vi "Update.vi"(8 "error in (no error)":errorcluster, 10 "Message in":refnum<class "UpdateMessage.lvclass">, 11 "ExampleClassB in":refnum<class "ExampleClassB.lvclass">) -> (0 "error out":errorcluster, 3 "ExampleClassB out":refnum<class "ExampleClassB.lvclass">)   [LabVIEW 2012, in "ExampleClassB.lvclass"]
doc: "The update method processes the command 'update'. \n\nThe command 'update' is used for receiving new values to be set to the private data of the class. This could be seen as a public set method for setting new parameters to the private class data."
uses:
  ExampleClassB.lvclass
  <vilib>/Distrio/Murmex/UpdateMessage/UpdateMessage.lvclass
  ExampleClassB.lvclass/ExampleClassB.ctl
  <vilib>/Distrio/Murmex/Murmex/status_enum.ctl
  <vilib>/Distrio/Murmex/Murmex/Murmex.lvclass
  <vilib>/Distrio/Murmex/Message/Message.lvclass
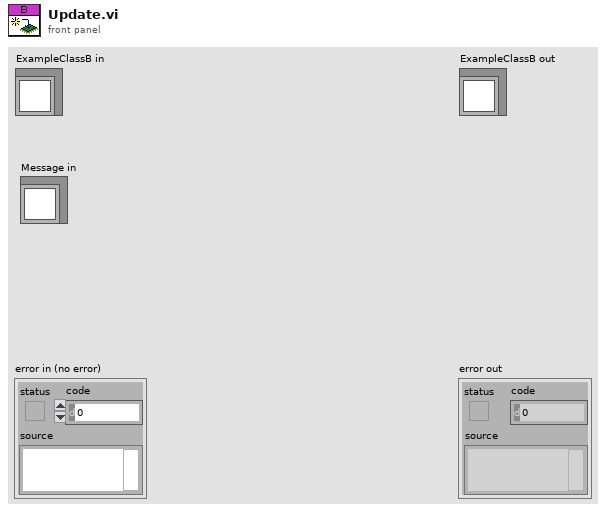
[diagram p1: front panel]
types:
  T1 = typedef "Murmex.lvlib/Murmex.lvclass/status_enum.ctl" = enum16{"ready", "warning", "error", "shutting down", "initialising"}
  T2 = typedef "ExampleClassB.lvclass/Settings cluster.ctl" = cluster{"expected samples":i32}
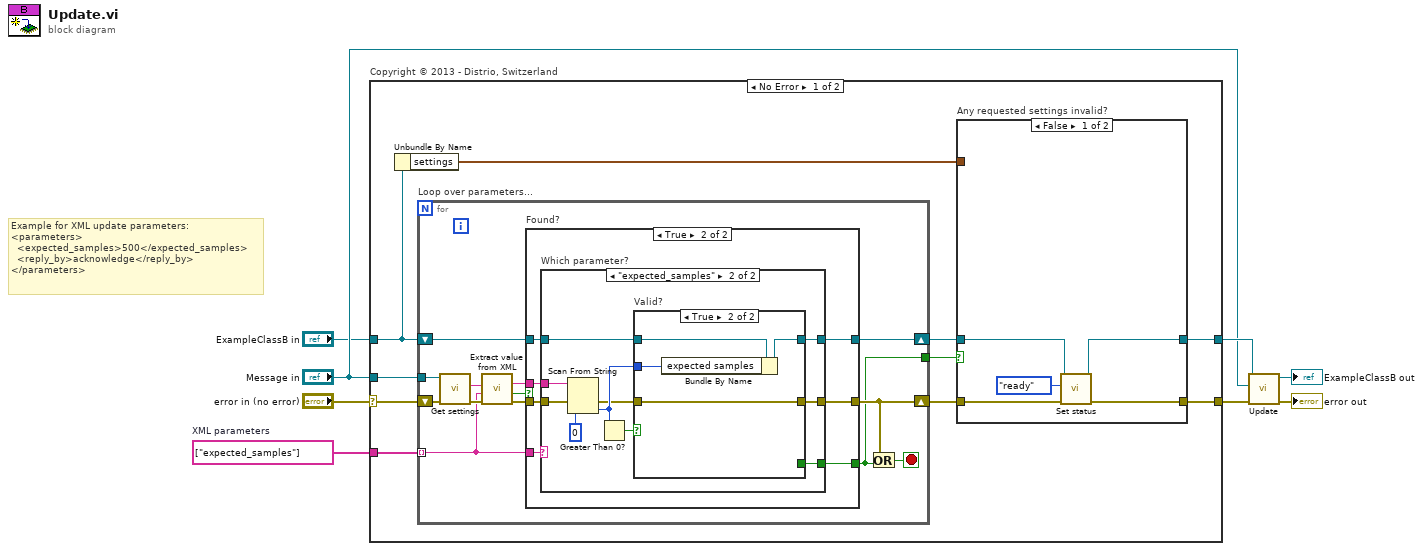
[diagram p0: block diagram]
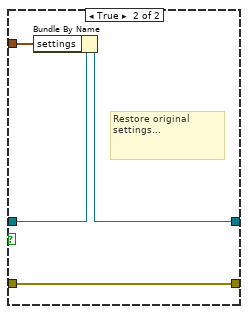
[diagram p2: hidden frame]
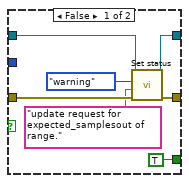
[diagram p5: hidden frame]
diagram:
  w8 = string[] ["expected_samples"]  # XML parameters
  # "Example for XML update parameters:\n<parameters>\n  <expected_samples>500</expected_samples>\n  <reply_by>acknowledge</reply_by>\n</parameters>"
  n1 = case "Copyright © 2013 - Distrio, Switzerland" shown="No Error" "error in (no error)" {
    selector: "error in (no error)" -> [w18 w73]
    tunnel: [w9 w73] -> w6
    tunnel: "ExampleClassB in" -> [w11 w74]
    tunnel: [w12 w74] -> w5
    tunnel: "Message in" -> [w17 _]
    tunnel: w8 -> [w16 _]
    frame No Error {
      n2 = Unbundle By Name(w11) -> ("settings"=w13:T2)
      n3 = for "Loop over parameters..." {
        shift-right: [w36] -> w10
        shift-left: w18 -> [w38]
        tunnel: w16 -> [w28] mode=indexing
        tunnel: w17 -> [w37]
        shift-right: [w39] -> w15
        shift-left: w11 -> [w40]
        tunnel: [w34] -> w14
        stop <- w35 stop-if-true
        n4 = call <vilib>:"Get settings.vi"("error in (no error)"=w38, "UpdateMessage in"=w37) -> ("error out"=w33:errorcluster, "settings"=w32:string)  [unwired: 7 in, 1 out]
        n5 = call <vilib>:"Extract value from XML.vi"("error in (no error)"=w33, "tag name"=w28, "parameters XML"=w32) -> ("error out"=w30:errorcluster, "found?"=w31:bool, "value"=w29:string)  [unwired: 5 in, 1 out]
        n6 = case "Found?" shown="True" w31 {
          tunnel: w30 -> [w42 w46]
          tunnel: [w42 w49] -> w36
          tunnel: w28 -> [_ w48]
          tunnel: w29 -> [_ w47]
          tunnel: w40 -> [w41 w45]
          tunnel: [w41 w44] -> w39
          tunnel: [_ w43] -> w34
          frame False {
          }
          frame True {
            n7 = case "Which parameter?" shown="\"expected_samples\"" w48 {
              tunnel: [w51 w54] -> w49
              tunnel: w47 -> [_ w57]
              tunnel: w46 -> [w51 w61]
              tunnel: w45 -> [w50 w59]
              tunnel: [w50 w58] -> w44
              tunnel: [_ w52] -> w43
              frame Default {
              }
              frame "expected_samples" {
                n8 = Scan From String(input string=w57, error in=w61, default 1=0) -> (error out=w55:errorcluster, output 1=w56:i32)  [unwired: 2 in, 2 out]
                n9 = Greater Than 0?(x=w56) -> (x > 0?=w53:bool)
                n10 = case "Valid?" shown="True" w53 {
                  tunnel: w59 -> [w68 w72]
                  tunnel: [w65 w71] -> w58
                  tunnel: w56 -> [_ w70]
                  tunnel: w55 -> [w67 w69]
                  tunnel: [w66 w69] -> w54
                  tunnel: [TRUE _] -> w52
                  frame False {
                    n11 = call <vilib>:"Set status.vi"("error in (no error)"=w67, "details"="update request for expected_samplesout of range.", "status"=status_enum."warning", "Murmex in"=w68) -> ("error out"=w66:errorcluster, "Murmex out"=w65:refnum<class "ExampleClassB.lvclass">)  [unwired: 6 in]
                  }
                  frame True {
                    n12 = Bundle By Name(cluster=w72, "expected samples"=w70) -> (w71:refnum<class "ExampleClassB.lvclass">)
                  }
                }
              }
            }
          }
        }
        n13 = Or(x=w36, y=w34) -> (x .or. y?=w35:bool)
      }
      n14 = case "Any requested settings invalid?" shown="False" w14 {
        tunnel: w15 -> [w21 w27]
        tunnel: w13 -> [_ w26]
        tunnel: [w20 w25] -> w12
        tunnel: w10 -> [w23 w24]
        tunnel: [w22 w24] -> w9
        frame False {
          n15 = call <vilib>:"Set status.vi"("error in (no error)"=w23, "status"=status_enum."ready", "Murmex in"=w21) -> ("error out"=w22:errorcluster, "Murmex out"=w20:refnum<class "ExampleClassB.lvclass">)  [unwired: 7 in]
        }
        frame True {
          # "Restore original settings..."
          n16 = Bundle By Name(cluster=w27, "settings"=w26) -> (w25:refnum<class "ExampleClassB.lvclass">)
        }
      }
    }
    frame Error {
    }
  }
  n17 = call-parent "Update.vi"("error in (no error)"=w6, "Message in"="Message in", "Murmex in"=w5) -> ("error out"=→"error out":errorcluster, "Murmex out"=→"ExampleClassB out":refnum<class "ExampleClassB.lvclass">)  [unwired: 7 in]
